vi "VI_Close.vi"(11 "VI_In":refnum<vi>) -> (3 "VI_Out":refnum<vi>)   [LabVIEW 2015]
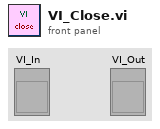
[diagram p1: front panel]
types:
  T1 = enum32{"Bad", "Idle", "Run top level", "Running"}
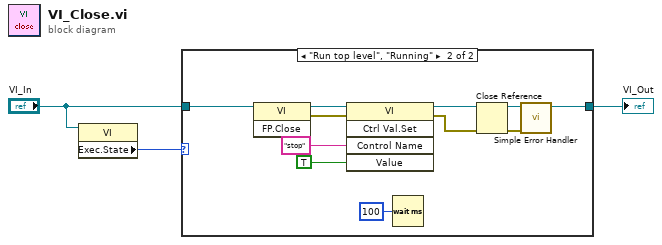
[diagram p0: block diagram]
diagram:
  n1 = property class="VI"(reference="VI_In") -> ("Exec.State"=w1:T1)  [unwired: 1 in, 2 out]
  n2 = case shown="\"Run top level\", \"Running\"" w1 {
    tunnel: [w4 w10] -> w3
    tunnel: "VI_In" -> [w4 w6]
    frame "Bad", Default {
    }
    frame "Run top level", "Running" {
      n3 = invoke class="VI" method="FP.Close"(reference=w6) -> (reference out=w13:refnum<vi>, error out=w12:errorcluster)  [unwired: 2 in, 1 out]
      n4 = invoke class="VI" method="Ctrl Val.Set"(reference=w13, error in=w12, "Control Name"="stop", "Value"=TRUE) -> (reference out=w10:refnum<vi>, error out=w9:errorcluster)  [unwired: 1 in, 3 out]
      n5 = Wait (ms)(milliseconds to wait=u32 100) -> ()  [unwired: 1 out]
      n6 = Close Reference(reference=w10, error in (no error)=w9) -> (error out=w8:errorcluster)
      n7 = call <vilib>:"Simple Error Handler.vi"("error in (no error)"=w8) -> ()  [unwired: 4 in, 5 out]
    }
  }
  "VI_Out" <- w3
